vi "Actor.vi"(5 "Alias":string, 6 "Creator Attributes":refnum<class "Attributes.lvclass">, 7 "Unified Msg Set":T1, 9 "Queue of Self Attributes":refnum<queue>, 10 "Queue of Error":refnum<queue>, 11 "Developer Utilities in":refnum<class "Developer Utilities.lvclass">) -> (0 "Error out":errorcluster, 3 "Developer Utilities out":refnum<class "Developer Utilities.lvclass">)   [LabVIEW 2020, in "jettl.lvlib" / "Developer Utilities.lvclass"]
uses:
  Developer Utilities.lvclass
  Attributes/Attributes/Attributes.lvclass
  Msg/Msg.lvclass
  Actor/Msg Set.ctl
  Actor/Actor.lvlib
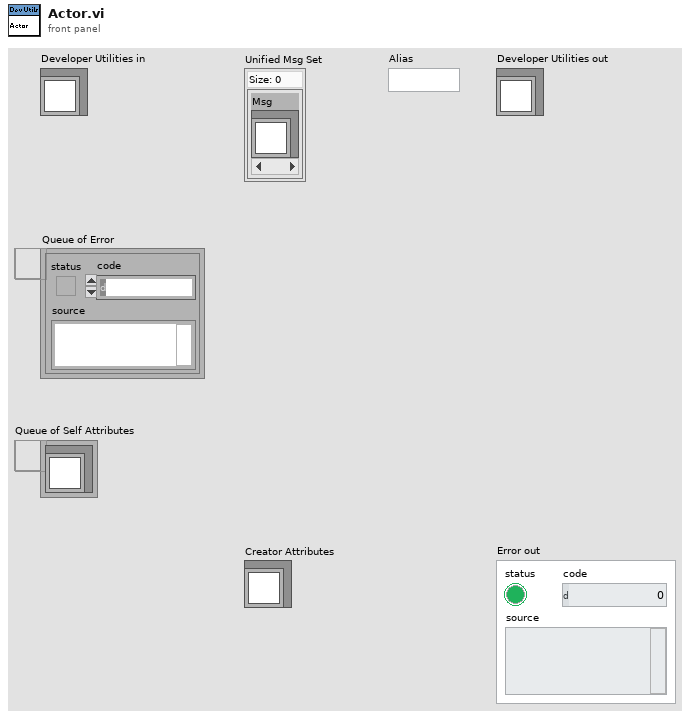
[diagram p1: front panel]
types:
  T1 = typedef "jettl.lvlib/Actor.lvlib/Msg Set.ctl" = set{refnum<class "Msg.lvclass">}
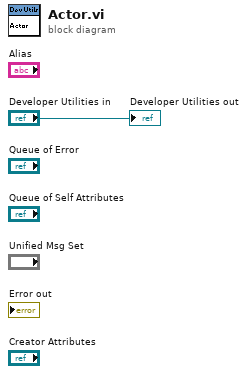
[diagram p0: block diagram]
diagram:
  "Developer Utilities out" <- "Developer Utilities in"
